vi "check HOLD and resend.vi"(8 "error in":errorcluster) -> (0 "error out 2":errorcluster)   [LabVIEW 2016]
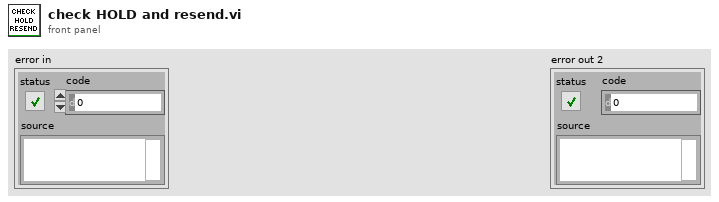
[diagram p1: front panel]
types:
  T1 = cluster{"Hold":bool, "Clamp":bool, "To Set":bool, "To Zero":bool, "Send to IPS":bool, "PS Heat":bool, "Lambda":bool}
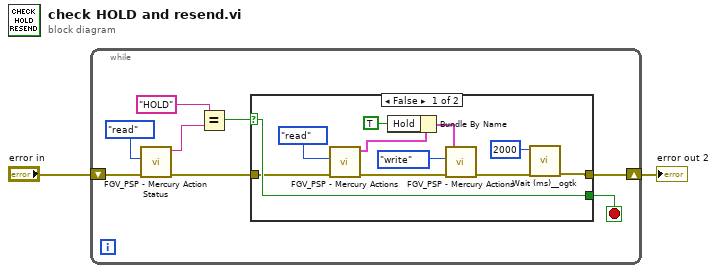
[diagram p0: block diagram]
diagram:
  n1 = while {
    shift-right: [w6] -> w1
    shift-left: "error in" -> [w3]
    stop <- w5 stop-if-true
    n2 = call "FGV_PSP - Mercury Action Status.vi"("error in"=w3, "Function"=enum16{"write", "read"}."read") -> ("error out"=w7:errorcluster, "Mercury Status 2"=w4:string)  [unwired: 4 in]
    n3 = Equal?(x="HOLD", y=w4) -> (x = y?=w8:bool)
    n4 = case shown="False" w8 {
      selector: w8 -> [w18 w22]
      tunnel: [w18 w22] -> w5
      tunnel: w7 -> [w16 w23]
      tunnel: [w11 w23] -> w6
      frame False {
        n5 = call "FGV_PSP - Mercury Actions.vi"("error in"=w16, "Function"=enum16{"write", "read"}."read") -> ("error out"=w15:errorcluster, "mercury actions 2"=w14:T1)  [unwired: 4 in]
        n6 = Bundle By Name(cluster=w14, "Hold"=TRUE ("Send to IPS")) -> (w21:T1)
        n7 = call "FGV_PSP - Mercury Actions.vi"("error in"=w15, "Function"=enum16{"write", "read"}."write", "mercury actions"=w21) -> ("error out"=w13:errorcluster)  [unwired: 3 in, 1 out]
        n8 = call <userlib>:"Wait (ms)__ogtk.vi"("error in (no error)"=w13, "milliseconds to wait"=u32 2000) -> ("error out"=w11:errorcluster)  [unwired: 8 in, 1 out]
      }
      frame True {
      }
    }
  }
  "error out 2" <- w1
